vi "19.3-FFTConverlution.vi"() -> ()   [LabVIEW 2020]
doc: "Uses the Median Filter VI to analyze pulses in the presence of noise. The example generates a pulse contaminated with Gaussian noise and applies a median filter. For comparison purposes, the VI computes the pulse parameters of the filtered pulse."
uses:
  <vilib>/Analysis/2dsp.llb/1D Convolution (DBL).vi
  <vilib>/Analysis/2dsp.llb/Real FFT.vi
  <vilib>/Analysis/2dsp.llb/Inverse Real FFT.vi
  <vilib>/Analysis/NI_AALBase.lvlib
  <vilib>/Analysis/NI_AALPro.lvlib
panel:
  out "x[n]*h[n]":dbl[](graph)
  out "x[n]":dbl[][](graph)
  out "h[t]":dbl[](graph) caption="h[n]"
  out "x[n]*h[n]":dbl[](graph)
  out "X[k]H[k]":dbl[](graph)
  out "H[k]":dbl[](graph)
  out "h[t]2":dbl[](graph) caption="h[n] (N+M+1)"
  out "X[k]":dbl[](graph)
  out "x[n]2":dbl[][](graph) caption="x[n] (N+M-1)"
  # "rFFT(X[k]H[k])"
  # "FFT(x[n])"
  # "FFT(h[n])"
  # "="
  # "X"
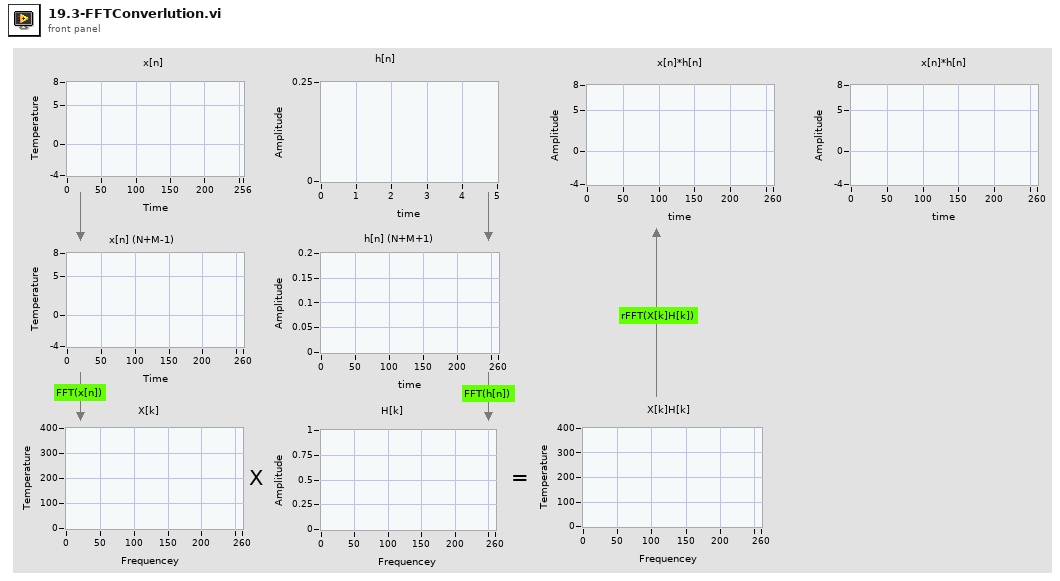
[diagram p1: front panel]
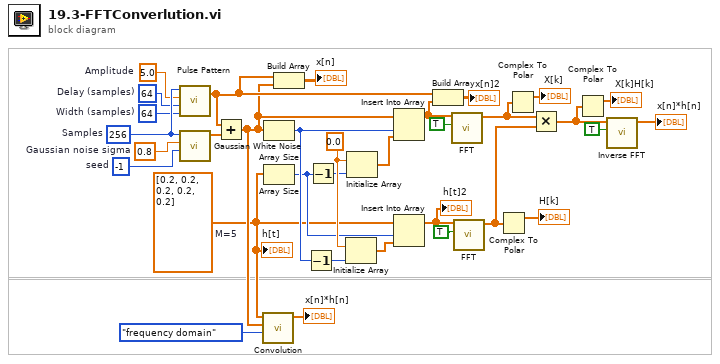
[diagram p0: block diagram]
diagram:
  w21 = 0.0 ("new element/subarray")
  w3 = dbl[] [0.2, 0.2, 0.2, 0.2, 0.2]  # M=5
  w33 = -1  # seed
  w32 = 0.8  # Gaussian noise sigma
  w28 = 64  # Width (samples)
  w29 = 64  # Delay (samples)
  w30 = 5.0  # Amplitude
  w31 = 256  # Samples
  n1 = call <vilib>:"Pulse Pattern.vi"("width"=w28, "delay"=w29, "amplitude"=w30, "samples"=w31) -> ("Pulse Pattern"=w11:dbl[])  [unwired: 1 out]
  n2 = call <vilib>:"Gaussian White Noise.vi"("seed"=w33, "standard deviation"=w32, "samples"=w31) -> ("Gaussian noise pattern"=w26:dbl[])  [unwired: 7 in, 1 out]
  n3 = Add(x=w11, y=w26) -> (x+y=w4:dbl[])
  n4 = call-poly <vilib>:"Convolution.vi"("algorithm"=enum32{"direct", "frequency domain"}."frequency domain", "Y"=w4, "X"=w3) -> ("X * Y"=→"x[n]*h[n]":dbl[])  [unwired: 7 in, 1 out]
  n5 = Array Size(array=w4) -> (size(s)=w7:i32)
  n6 = Array Size(array=w3) -> (size(s)=w6:i32)
  n7 = Build Array(w11, w4) -> (→"x[n]":dbl[][])
  n8 = Decrement(x=w7) -> (x-1=w8:i32)
  n9 = Decrement(x=w6) -> (x-1=w9:i32)
  n10 = Initialize Array(w21, w8) -> (w22:dbl[])
  n11 = Initialize Array(w21, w9) -> (w23:dbl[])
  n12 = Insert Into Array(array=w4, index=w7, new element=w23) -> (w10:dbl[])
  n13 = Insert Into Array(array=w3, index=w6, new element=w22) -> (w20:dbl[])
  "h[t]2" <- w20
  n14 = Build Array(w11, w10) -> (→"x[n]2":dbl[][])
  n15 = call-poly <vilib>:"FFT.vi"("shift?"=TRUE, "X"=w10) -> ("FFT {X}"=w19:cdb[])  [unwired: 8 in, 1 out]
  n16 = call-poly <vilib>:"FFT.vi"("shift?"=TRUE, "X"=w20) -> ("FFT {X}"=w17:cdb[])  [unwired: 8 in, 1 out]
  n17 = Complex To Polar(r * e^(i*theta)=w17) -> (r=→"H[k]":dbl[])  [unwired: 1 out]
  n18 = Complex To Polar(r * e^(i*theta)=w19) -> (r=→"X[k]":dbl[])  [unwired: 1 out]
  n19 = Multiply(x=w19, y=w17) -> (x*y=w14:cdb[])
  n20 = Complex To Polar(r * e^(i*theta)=w14) -> (r=→"X[k]H[k]":dbl[])  [unwired: 1 out]
  n21 = call-poly <vilib>:"Inverse FFT.vi"("shift?"=TRUE, "FFT {X}"=w14) -> ("X"=→"x[n]*h[n]":dbl[])  [unwired: 8 in, 1 out]
  "h[t]" <- w3
